vi "PDF Konfig Dichtheitstest.vi"(8 "error in (no error)":errorcluster caption="Fehler (Eingang, kein Fehler)", 11 "seconds since 1Jan1904":timestamp) -> (0 "error out":errorcluster caption="Fehler (Ausgang)", 3 "PDF Pfad":path)   [LabVIEW 2020, in "Erweiterte Konfig.lvlib"]
uses:
  Erweiterte Konfig.lvlib
  Schedule Modul/Aktion FGV Testdaten sammeln.ctl
  Sprachverwaltung/FGV Aktion Tabelle zerlegen.ctl
  Linearisierung V2/Protokoll/Protokoll.lvlib
  Schedule Modul/Schedule Modul.lvlib
  Sprachverwaltung/Sprachverwaltung.lvlib
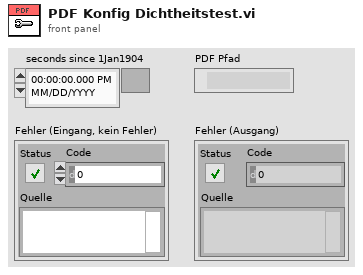
[diagram p1: front panel]
types:
  T1 = typedef "Sprachverwaltung.lvlib/FGV Aktion Tabelle zerlegen.ctl" = enum16{"laden", "vereinzeln", "speichern"}
  T2 = typedef "Schedule Modul.lvlib/Aktion FGV Testdaten sammeln.ctl" = enum16{"lesen", "Dichtheitstest", "CalGasTest", "T90", "Kalibrieren", "init", "Kalender Daten"}
  T3 = typedef "Schedule Modul.lvlib/Ergebnis Dichtheitstest.ctl" = cluster{"Druck FT-IR:":T4, "max. Anstieg:":T4, "Druckanstieg:":T4, "Zeitdauer:":T4, "Verstrichene Zeit:":T4, "Fehler":bool, "Unterdruck nicht erreicht ":bool}
  T4 = typedef "Zahlen-Ausgabefeld.ctl" = sgl
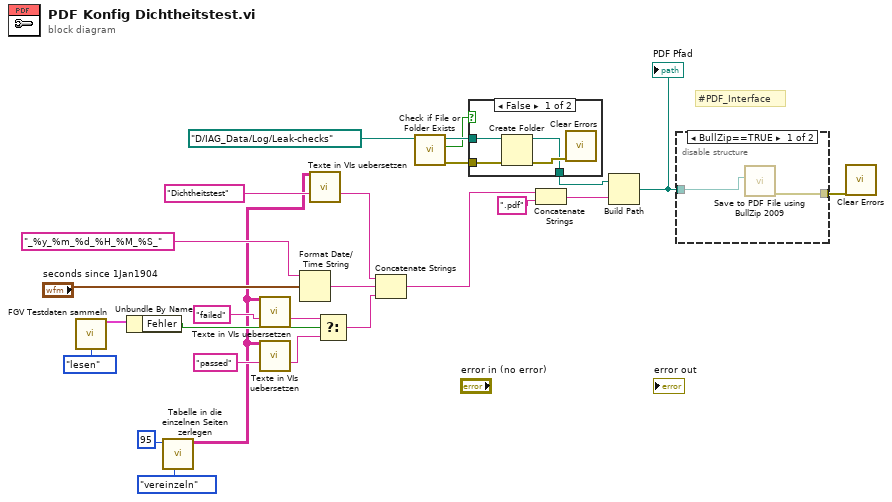
[diagram p0: block diagram]
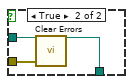
[diagram p2: hidden frame]
diagram:
  # "#PDF_Interface"
  n1 = call "FGV Testdaten sammeln.vi"("Aktion"=Aktion_FGV_Testdaten_sammeln."lesen") -> ("Ergebnisse Dichtheitstest"=w17:T3)  [unwired: 9 in, 5 out]
  n2 = Unbundle By Name(w17) -> ("Fehler"=w18:bool)
  n3 = call "Tabelle in die einzelnen Seiten zerlegen.vi"("Aktion"=FGV_Aktion_Tabelle_zerlegen."vereinzeln", "Index (Seite)"=95) -> ("Sprachliste"=w1:string[][])  [unwired: 7 in, 2 out]
  n4 = call "Texte in VIs uebersetzen.vi"("Sprachliste"=w1, "String zum Übersetzen"="failed" ("String")) -> ("String zum Übersetzen"=w3:string)  [unwired: 9 in, 4 out]
  n5 = call "Texte in VIs uebersetzen.vi"("Sprachliste"=w1, "String zum Übersetzen"="passed" ("String")) -> ("String zum Übersetzen"=w2:string)  [unwired: 9 in, 4 out]
  n6 = Format Date/Time String(time format string (%c)="_%y_%m_%d_%H_%M_%S_" ("Zeitformatierungs-String (%c)"), seconds (now)="seconds since 1Jan1904") -> (date/time string=w14:string)  [unwired: 1 in]
  n7 = call "Texte in VIs uebersetzen.vi"("Sprachliste"=w1, "String zum Übersetzen"="Dichtheitstest" ("String")) -> ("String zum Übersetzen"=w7:string)  [unwired: 9 in, 4 out]
  n8 = Select(t=w3, s=w18, f=w2) -> (s? t:f=w6:string)
  n9 = Concatenate Strings(w7, w14, w6) -> (w19:string)
  n10 = call <vilib>:"Check if File or Folder Exists.vi"("path"=path "D:/IAG_Data/Log/Leak-checks" ("Pfad:")) -> ("error out"=w26:errorcluster, "file or folder exists?"=w23:bool, "dup path"=w24:path)  [unwired: 8 in]
  n11 = case shown="False" w23 {
    tunnel: w24 -> [w30 w32]
    tunnel: [w28 w32] -> w25
    tunnel: w26 -> [w27 w31]
    frame False {
      n12 = Create Folder(path (use dialog)=w30, error in=w27) -> (created path=w28:path, error out=w29:errorcluster)  [unwired: 1 in, 1 out]
      n13 = call <vilib>:"Clear Errors.vi"("error in (no error)"=w29) -> ()  [unwired: 5 in, 2 out]
    }
    frame True {
      n14 = call <vilib>:"Clear Errors.vi"("error in (no error)"=w31) -> ()  [unwired: 5 in, 2 out]
    }
  }
  n15 = Concatenate Strings(w19, ".pdf" ("String")) -> (w11:string)
  n16 = Build Path(base path=w25, name or relative path=w11) -> (appended path=w20:path)
  "PDF Pfad" <- w20
  n17 = disable-structure shown="BullZip==TRUE" {
    disable-tunnel: [w34 _] -> w21
    disable-tunnel: w20 -> [w33 _]
    frame condition #0 {
      n18 = call "Save to PDF File using BullZip 2009.vi"("Save PDF File Path"=w33) -> ("error out"=w34:errorcluster)  [unwired: 10 in]
    }
    frame condition #1 (active) {
    }
  }
  n19 = call <vilib>:"Clear Errors.vi"("error in (no error)"=w21) -> ()  [unwired: 5 in, 2 out]
